vi "Alazar module U16.vi"(3 "Imag window array":sgl[](array[numeric]), 4 "Acq Settings":T2={"Window Type"=1, "Record Length"=1536, "Footer"=0, "Offset"=0, "Records Per Buffer"=1000, "Samples per record"=2048, "Records Count (Records/Acq)"=2147483647, "Output Format"=11} {"Output Format" items=["U16_LOG"=1, "U16_AMP2"=257]; "Window Type" items=["DSP_WINDOW_NONE", "DSP_WINDOW_HANNING", "DSP_WINDOW_HAMMING", "DSP_WINDOW_BLACKMAN", "DSP_WINDOW_BLACKMAN_HARRIS", "DSP_WINDOW_BARTLETT"]; "Footer" items=["FOOTER_NONE", "FOOTER_NPT"]}, 5 "Channel":u32(ring)=1 items=["A"=1, "B"=2, "A + B"=3, "C"=4, "A + C"=5, "A + B"=6, "D"=8, "A + D"=9, "B + D"=10, "C + D"=12, "A + B + C + D"=15], 6 "Trigger Settings":T5={"General Trigger Settings"={"Trigger Operation"=0, "Coupling ID"=2, "Range ID"=0, "Delay"=0, "Timeout Ticks"=0, "Mode"=0, "Parameter"=0}, "Trigger Engine 1"={"Trigger Engine"=0, "Source"=0, "Slope"=1, "Level"=0}, "Trigger Engine 2"={"Trigger Engine"=0, "Source"=0, "Slope"=1, "Level"=0}} {"General Trigger Settings"."Trigger Operation" items=["J", "K", "J OR K", "J AND K", "J XOR K", "J AND NOT K", "NOT J AND K"]; "General Trigger Settings"."Coupling ID" items=["AC"=1, "DC"=2]; "General Trigger Settings"."Range ID" items=["5 V", "1 V", "TTL"]; "Trigger Engine 1"."Trigger Engine" items=["J", "K"]; "Trigger Engine 1"."Source" items=["A", "B", "External", "Disable", "C", "D"]; "Trigger Engine 1"."Slope" items=["Positive"=1, "Negative"=2]; "Trigger Engine 2"."Trigger Engine" items=["J", "K"]; "Trigger Engine 2"."Source" items=["A", "B", "External", "Disable", "C", "D"]; "Trigger Engine 2"."Slope" items=["Positive"=1, "Negative"=2]}, 7 "Action":T1=enum."Config Trig", 8 "error in (no error)":errorcluster, 9 "Ch Input Control":T6={"Channel"=1, "Coupling"=2, "Range"=10, "Impedance"=2} {"Channel" items=["A"=1, "B"=2, "C"=4, "D"=8]; "Coupling" items=["AC"=1, "DC"=2]; "Range" items=["20 mV"=1, "40 mV"=2, "50 mV"=3, "80 mV"=4, "100 mV"=5, "200 mV"=6, "400 mV"=7, "500 mV"=8, "800 mV"=9, "1 V"=10, "1.25 V"=33, "2 V"=11, "4 V"=12, "5 V"=13, "8 V"=14, "10 V"=15, "20 V"=16]; "Impedance" items=["1 MOhm"=1, "50 Ohm"=2, ""=0]}, 10 "Capture Clock":T7={"Sample Rate"=30, "Decimation"=0, "Source"=1, "Edge"=0} {"Edge" items=["Rising", "Falling"]; "Source" items=["Internal"=1, "Fast External"=2, "Medium External"=3, "Slow External"=4, "External AC"=5, "External DC"=6, "External 10MHz"=7]}, 11 "Device ID":T8={"System ID"=1, "Board ID"=1}) -> (0 "error out":errorcluster, 1 "Return Code":u32, 2 "Buffer":u16[](array[numeric]))   [LabVIEW 2018]
uses:
  Hardware Mfg/AlazarTech SDK/Controls/Alazar Device ID.ctl
  Hardware Mfg/AlazarTech SDK/Controls/Clock Controls.ctl
  Hardware Mfg/AlazarTech SDK/Controls/Channel Input Controls.ctl
  Hardware Mfg/AlazarTech SDK/Controls/General Trigger Settings.ctl
  Hardware Mfg/AlazarTech SDK/Controls/Trigger Engine Controls.ctl
  Hardware Mfg/AlazarTech SDK/Controls/Alazar Acquisition Settings.ctl
  Hardware Mfg/AlazarTech SDK/Controls/Alazar Engine Actions.ctl
  Hardware Mfg/AlazarTech SDK/Controls/Async Read Parameters.ctl
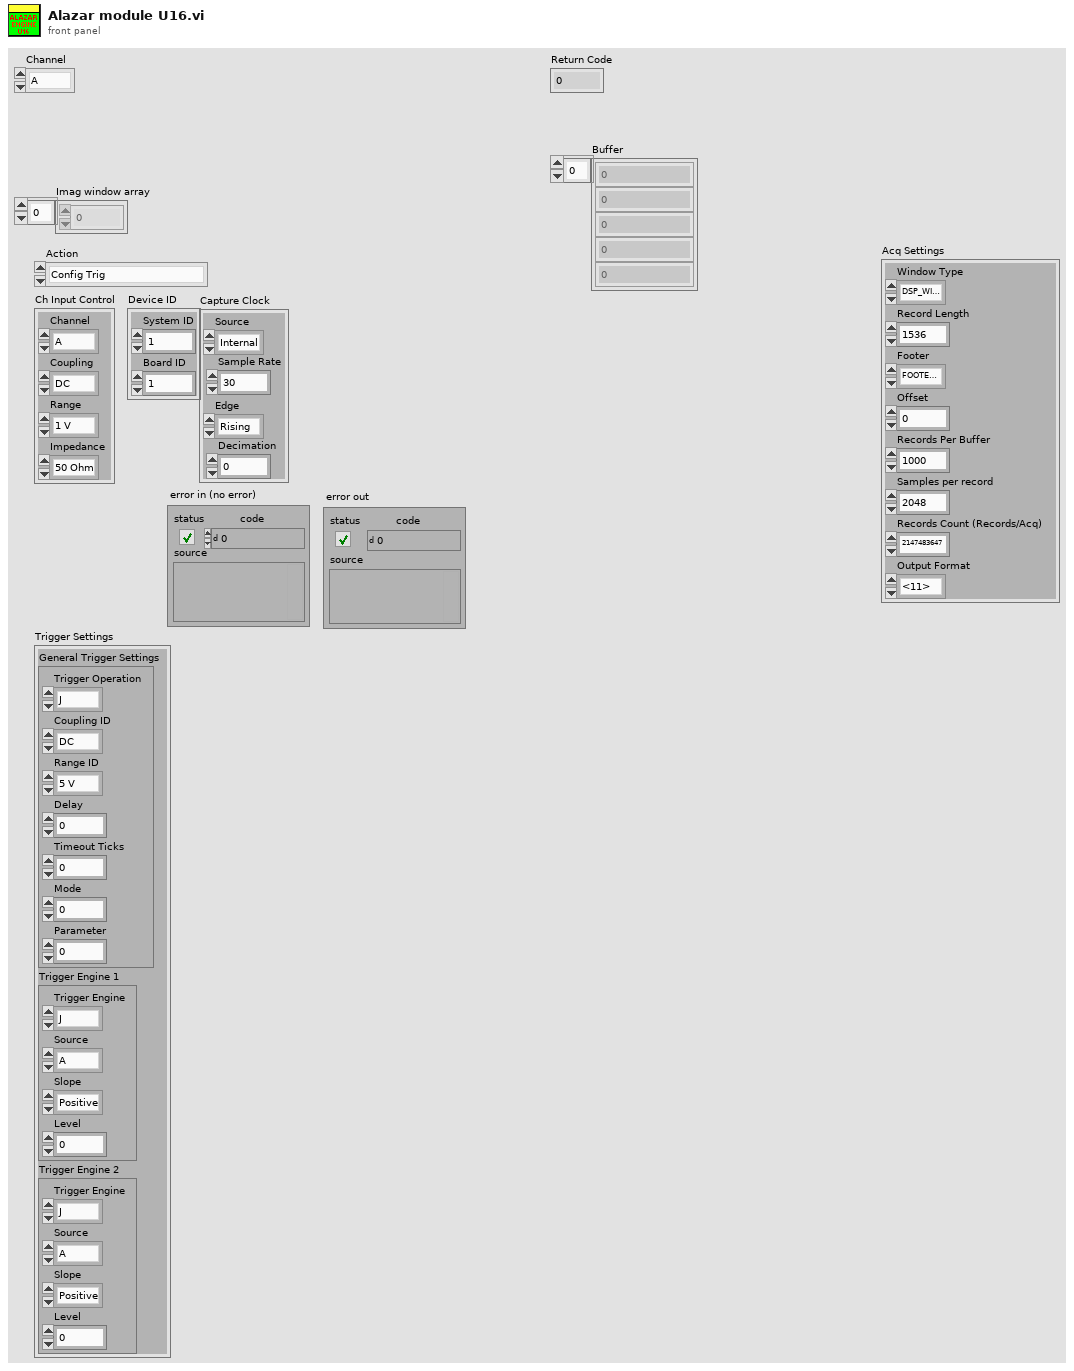
[diagram p1: front panel]
types:
  T1 = typedef "Alazar Engine Actions.ctl" = enum16{"Init", "Config Clock", "Config Ch", "Config Trig", "Config Non-FFT Acq.", "Non-FFT Acquire", "Load background from Non-FFT buffer", "enable background subtrac", "disable background subtrac", "load background from file", "load background from elsewhere", "start acquire", "background subtraction", "Config Acq.", "Acquire", "UnInit"}
  T2 = typedef "Alazar Acquisition Settings.ctl" = cluster{"Window Type":u32, "Record Length":u32, "Footer":u32, "Offset":u32, "Records Per Buffer":u32, "Samples per record":u32, "Records Count (Records/Acq)":u32, "Output Format":u32}
  T3 = typedef "General Trigger Settings.ctl" = cluster{"Trigger Operation":u32, "Coupling ID":u32, "Range ID":u32, "Delay":u32, "Timeout Ticks":u32, "Mode":u32, "Parameter":u32}
  T4 = typedef "Trigger Engine Controls.ctl" = cluster{"Trigger Engine":u32, "Source":u32, "Slope":u32, "Level":u32}
  T5 = cluster{"General Trigger Settings":T3, "Trigger Engine 1":T4, "Trigger Engine 2":T4}
  T6 = typedef "Channel Input Controls.ctl" = cluster{"Channel":u8, "Coupling":u32, "Range":u32, "Impedance":u32}
  T7 = typedef "Clock Controls.ctl" = cluster{"Sample Rate":u32, "Decimation":u32, "Source":u32, "Edge":u32}
  T8 = typedef "Alazar Device ID.ctl" = cluster{"System ID":u32, "Board ID":u32}
  T9 = typedef "Async Read Parameters.ctl" = cluster{"Transfer Offset":u32, "Transfer Length":u32, "Records Per Buffer":u32, "Records Per Acquisition":u32}
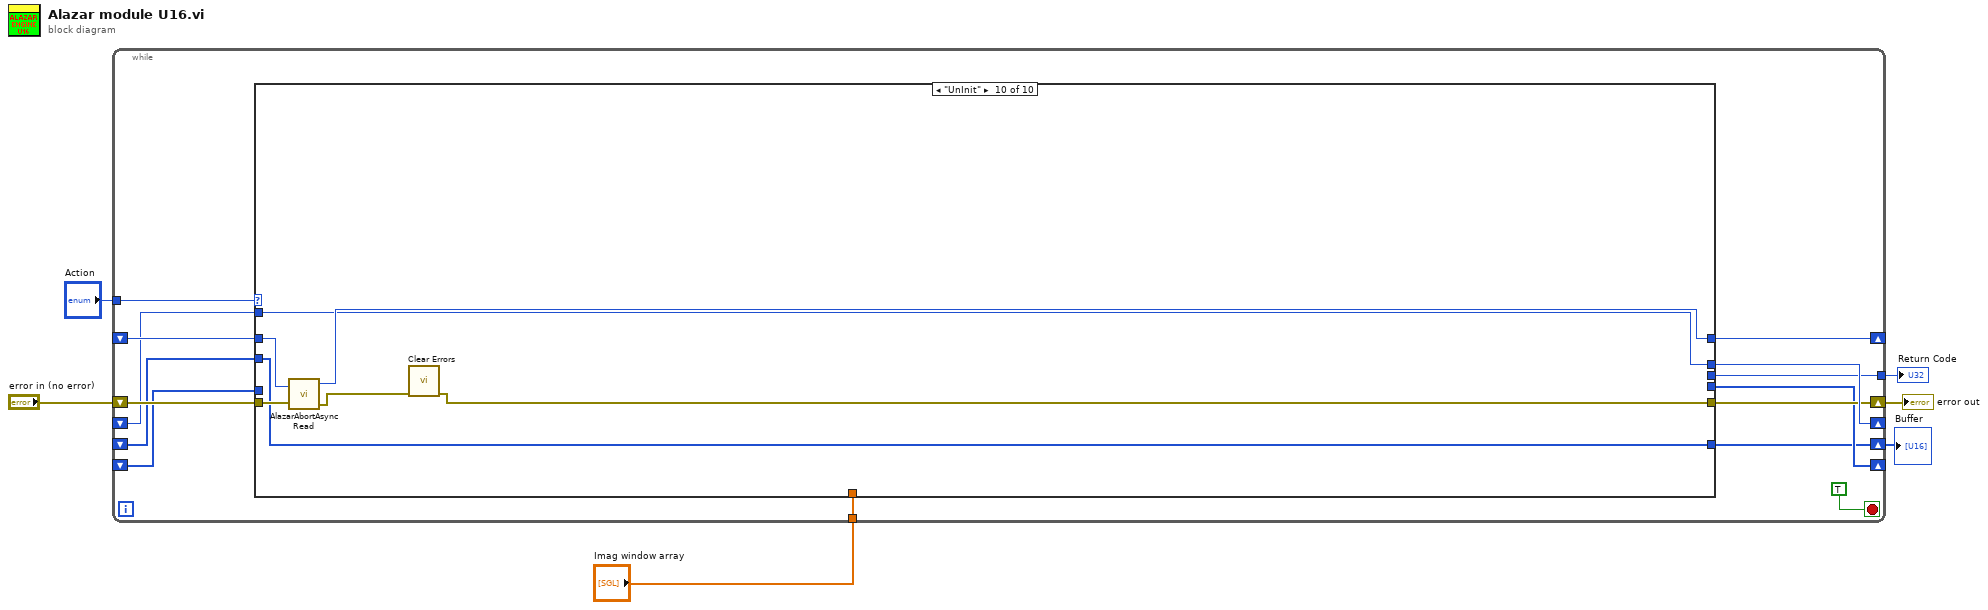
[diagram p0: block diagram]
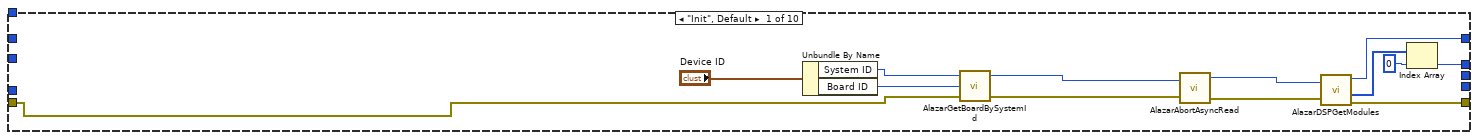
[diagram p2: hidden frame]
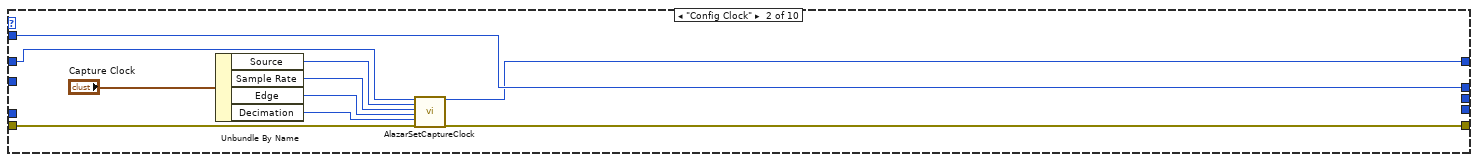
[diagram p3: hidden frame]
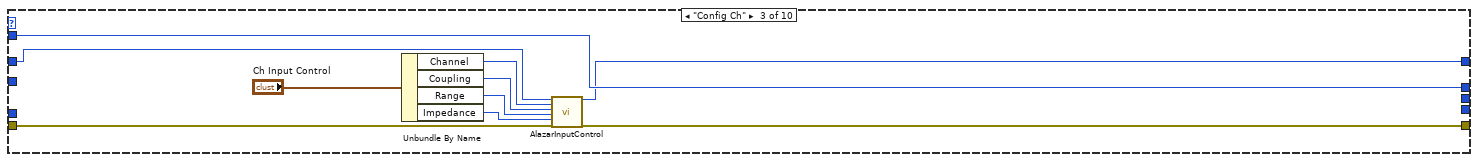
[diagram p4: hidden frame]
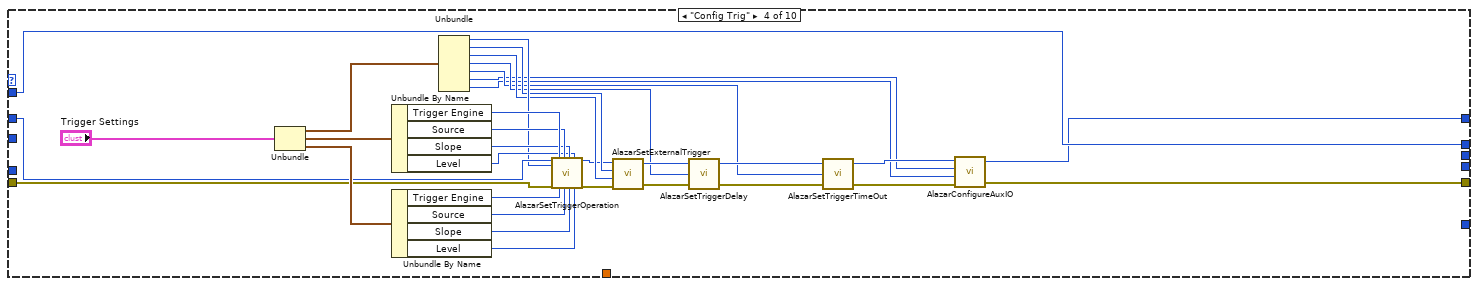
[diagram p5: hidden frame]
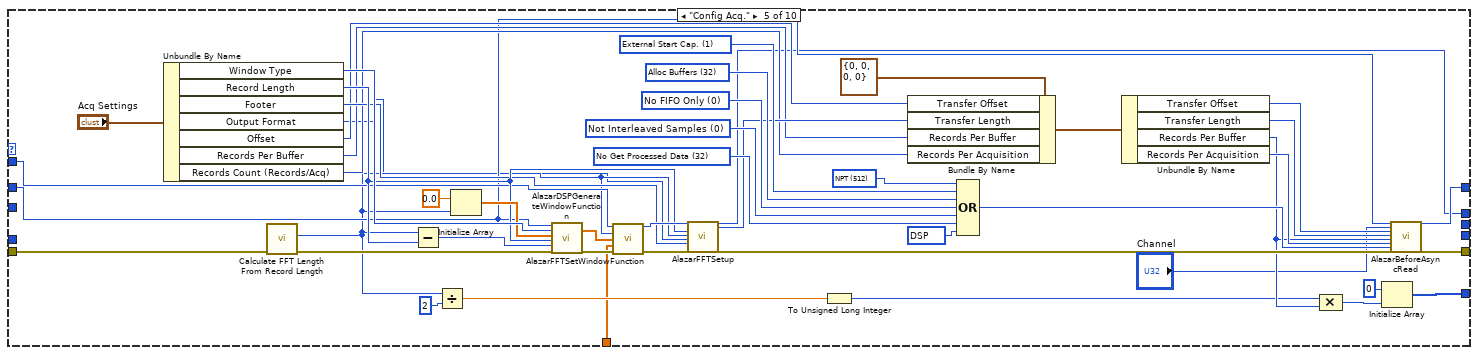
[diagram p6: hidden frame]
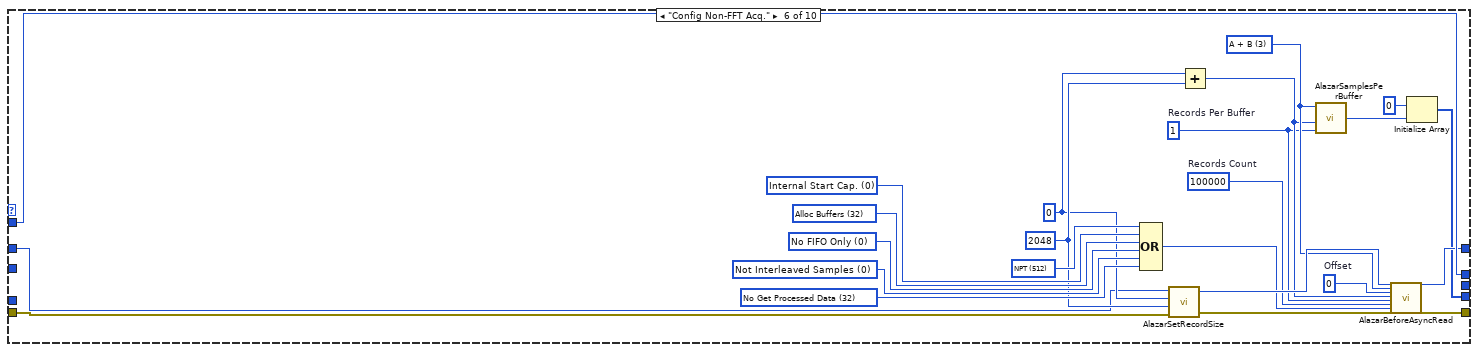
[diagram p7: hidden frame]
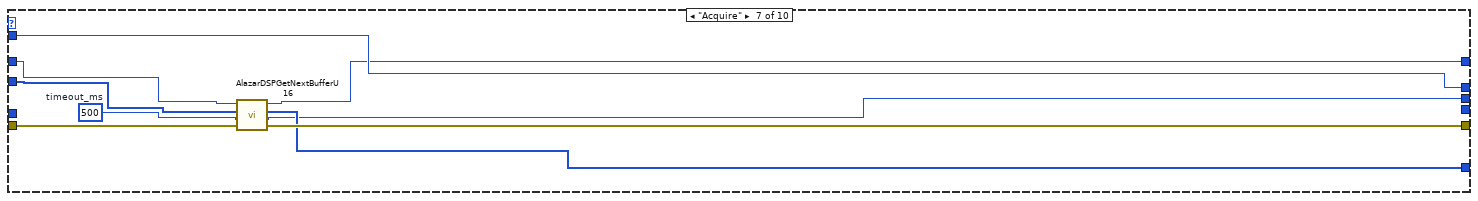
[diagram p8: hidden frame]
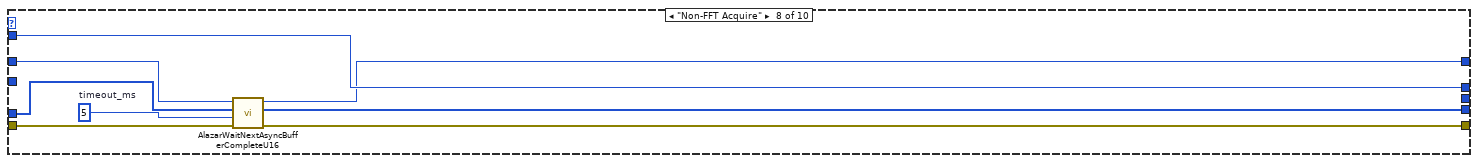
[diagram p9: hidden frame]
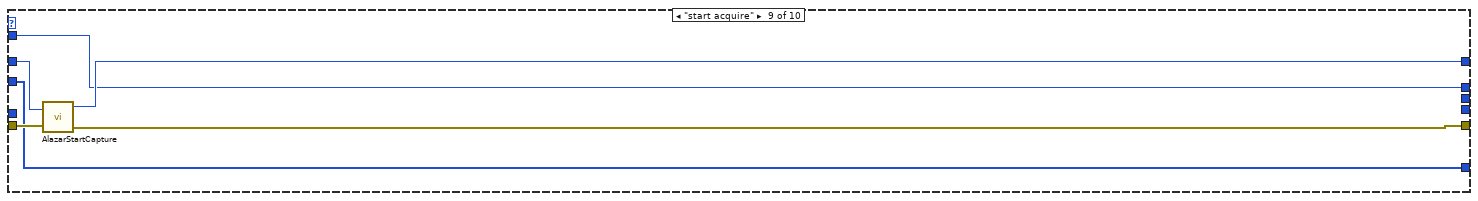
[diagram p10: hidden frame]
diagram:
  n1 = while {
    tunnel: "Action" -> [w18]
    shift-right: [w17] -> _
    shift-left: _ -> [w16]
    shift-right: [w15] -> _
    shift-left: _ -> [w14]
    shift-right: [w13] -> w4
    shift-left: "error in (no error)" -> [w19]
    shift-right: [w7] -> w1
    shift-left: _ -> [w12]
    shift-right: [w11] -> _
    shift-left: _ -> [w10]
    tunnel: "Imag window array" -> [w9]
    tunnel: [w8] -> w2
    stop <- TRUE stop-if-true
    n2 = case shown="\"UnInit\"" w18 {
      tunnel: w19 -> [w21 w41 w47 w67 w124 w138 w163 w170 w179 w186]
      tunnel: [w24 w34 w46 w55 w90 w137 w164 w167 w178 w180] -> w13
      tunnel: [w22 w35 w45 w54 w100 w134 w159 w168 w176 w184] -> w17
      tunnel: w16 -> [_ w36 w44 w72 w105 w136 w160 w171 w177 w185]
      tunnel: [w32 w43 w53 w83 w98 w135 w165 w169 w175 w183] -> w15
      tunnel: w14 -> [_ w43 w53 w83 w112 w135 w165 w169 w175 w183]
      tunnel: w12 -> [_ _ _ _ _ _ w161 _ w174 w181]
      tunnel: [_ _ _ _ _ w133 _ w166 _ _] -> w11
      tunnel: w10 -> [_ _ _ _ _ _ _ w172 _ _]
      tunnel: w9 -> [_ _ _ _ w88 _ _ _ _ _]
      tunnel: [_ _ _ _ _ _ w157 _ _ _] -> w8
      tunnel: [_ _ _ _ w87 _ w158 _ w174 w181] -> w7
      frame "Init", Default {
        n3 = Unbundle By Name("Device ID") -> ("System ID"=w30:u32, "Board ID"=w29:u32)
        n4 = call "AlazarGetBoardBySystemId.vi"("error in (no error)"=w21, "Board ID"=w29, "System ID"=w30) -> ("error out"=w28:errorcluster, "Handle"=w27:u64)  [unwired: 1 out]
        n5 = call "AlazarAbortAsyncRead.vi"("Handle"=w27, "error in (no error)"=w28) -> ("Handle"=w26:u64, "error out"=w25:errorcluster)  [unwired: 1 out]
        n6 = call "AlazarDSPGetModules.vi"("Handle"=w26, "error in (no error)"=w25) -> ("Handle"=w22:u64, "DSP Modules"=w23:u64[], "error out"=w24:errorcluster)  [unwired: 1 out]
        n7 = Index Array(array=w23, index=u32 0) -> (element=w32:u64)
      }
      frame "Config Clock" {
        n8 = Unbundle By Name("Capture Clock") -> ("Source"=w37:u32, "Sample Rate"=w38:u32, "Edge"=w39:u32, "Decimation"=w40:u32)
        n9 = call "AlazarSetCaptureClock.vi"("Handle"=w36, "Source"=w37, "Sample Rate"=w38, "Edge"=w39, "Decimation"=w40, "error in (no error)"=w41) -> ("Handle"=w35:u64, "error out"=w34:errorcluster)  [unwired: 11 in, 1 out]
      }
      frame "Config Ch" {
        n10 = Unbundle By Name("Ch Input Control") -> ("Channel"=w51:u8, "Coupling"=w50:u32, "Range"=w49:u32, "Impedance"=w48:u32)
        n11 = call "AlazarInputControl.vi"("Handle"=w44, "Channel"=w51, "Coupling"=w50, "Range"=w49, "Impedance"=w48, "error in (no error)"=w47) -> ("Handle"=w45:u64, "error out"=w46:errorcluster)  [unwired: 11 in, 1 out]
      }
      frame "Config Trig" {
        n12 = Unbundle("Trigger Settings") -> ("General Trigger Settings"=w84:T3, "Trigger Engine 1"=w82:T4, "Trigger Engine 2"=w81:T4)
        n13 = Unbundle By Name(w82) -> ("Trigger Engine"=w80:u32, "Source"=w79:u32, "Slope"=w78:u32, "Level"=w77:u32)
        n14 = Unbundle By Name(w81) -> ("Trigger Engine"=w76:u32, "Source"=w75:u32, "Slope"=w74:u32, "Level"=w73:u32)
        n15 = Unbundle(w84) -> ("Trigger Operation"=w71:u32, "Coupling ID"=w70:u32, "Range ID"=w69:u32, "Delay"=w63:u32, "Timeout Ticks"=w60:u32, "Mode"=w57:u32, "Parameter"=w56:u32)
        n16 = call "AlazarSetTriggerOperation.vi"("Handle"=w72, "Trigger Operation"=w71, "error in (no error)"=w67, "Trigger Engine 1"=w80, "Trigger Engine 2"=w76, "Source 1"=w79, "Source 2"=w75, "Slope 1"=w78, "Slope 2"=w74, "Level 1"=w77, "Level 2"=w73) -> ("Handle"=w65:u64, "error out"=w68:errorcluster)  [unwired: 6 in, 1 out]
        n17 = call "AlazarSetExternalTrigger.vi"("error in (no error)"=w68, "Range ID"=w69, "Coupling ID"=w70, "Handle"=w65) -> ("error out"=w66:errorcluster, "Handle"=w64:u64)  [unwired: 1 out]
        n18 = call "AlazarSetTriggerDelay.vi"("error in (no error)"=w66, "Delay"=w63, "Handle"=w64) -> ("error out"=w62:errorcluster, "Handle"=w61:u64)  [unwired: 1 out]
        n19 = call "AlazarSetTriggerTimeOut.vi"("error in (no error)"=w62, "Timeout Ticks"=w60, "Handle"=w61) -> ("error out"=w59:errorcluster, "Handle"=w58:u64)  [unwired: 1 out]
        n20 = call "AlazarConfigureAuxIO.vi"("error in (no error)"=w59, "Parameter"=w56, "Mode"=w57, "Handle"=w58) -> ("error out"=w55:errorcluster, "Handle"=w54:u64)  [unwired: 1 out]
      }
      frame "Config Acq." {
        w125 = u32 16384 items=["DSP"=16384]
        w131 = u32 32 items=["No Get Processed Data"=32, "Get Processed Data"=8192]
        w130 = u32 0 items=["Not Interleaved Samples"=0, "Interleave Samples"=4096]
        w126 = u32 0 items=["No FIFO Only"=0, "FIFO Only"=2048]
        w129 = u32 32 items=["Alloc Buffers"=32]
        w128 = u32 1 items=["Internal Start Cap.", "External Start Cap."]
        w127 = u32 512 items=["Traditional"=0, "NPT"=512, "Continuous"=256, "Triggered Streaming"=1024]
        n21 = Unbundle By Name("Acq Settings") -> ("Window Type"=w121:u32, "Record Length"=w115:u32, "Footer"=w114:u32, "Output Format"=w86:u32, "Offset"=w110:u32, "Records Per Buffer"=w108:u32, "Records Count (Records/Acq)"=w107:u32)
        n22 = call "Calculate FFT Length From Record Length.vi"("error in (no error)"=w124) -> ("error out"=w122:errorcluster, "FFT Length"=w96:u32)  [unwired: 8 in, 1 out]
        n23 = Subtract(x=w96, y=w115) -> (x-y=w120:u32)
        n24 = Divide(x=w96, y=u32 2) -> (x/y=w92:dbl)
        n25 = Initialize Array(sgl 0.0, w96) -> (w118:sgl[])
        n26 = call "AlazarDSPGenerateWindowFunction.vi"("Handle"=w105, "Window Type"=w121, "window"=w118, "WindowLength_samples"=w115, "PaddingLength_samples"=w120, "error in (no error)"=w122) -> ("window"=w119:sgl[], "error out"=w117:errorcluster)  [unwired: 10 in, 2 out]
        n27 = call "AlazarFFTSetWindowFunction.vi"("DSP Handle"=w112, "Samples per record"=w96, "Real window array"=w119, "Imag window array"=w88, "error in (no error)"=w117) -> ("DSP Handle"=w116:u64, "error out"=w113:errorcluster)  [unwired: 9 in]
        n28 = call "AlazarFFTSetup.vi"("DSP Handle"=w116, "Record Length (samples)"=w115, "FFT Length (samples)"=w96, "Output Format"=w86, "Footer"=w114, "error in (no error)"=w113) -> ("DSP Handle"=w98:u64, "Bytes Per Output Record"=w109:u32, "error out"=w99:errorcluster)  [unwired: 18 in, 1 out]
        n29 = To Unsigned Long Integer(number=w92) -> (unsigned 32bit integer=w91:u32)
        n30 = Bundle By Name(cluster=T9 {"Transfer Offset"=0, "Transfer Length"=0, "Records Per Buffer"=0, "Records Per Acquisition"=0} ("ASync Read Parameters"), "Transfer Offset"=w110, "Transfer Length"=w109, "Records Per Buffer"=w108, "Records Per Acquisition"=w107) -> (w106:T9)
        n31 = Compound Arithmetic op=OR(w127, w128, w129, w126, w130, w131, w125) -> (w101:u32)
        n32 = Unbundle By Name(w106) -> ("Transfer Offset"=w104:u32, "Transfer Length"=w103:u32, "Records Per Buffer"=w97:u32, "Records Per Acquisition"=w102:u32)
        n33 = Compound Arithmetic op=MULTIPLY(w91, w97) -> (w95:u32)
        n34 = Initialize Array(u16 0 ("element"), w95) -> (w87:u16[])
        n35 = call "AlazarBeforeAsyncRead.vi"("Handle"=w105, "Channel Select"="Channel", "Transfer Offset"=w104, "Transfer Length"=w103, "Records Per Buffer"=w97, "Records Per Acquisition"=w102, "Flags"=w101, "error in (no error)"=w99) -> ("Handle"=w100:u64, "error out"=w90:errorcluster)  [unwired: 17 in, 1 out]
      }
      frame "Config Non-FFT Acq." {
        w141 = u32 3 items=["A"=1, "B"=2, "A + B"=3, "C"=4, "A + C"=5, "A + B"=6, "D"=8, "A + D"=9, "B + D"=10, "C + D"=12, "A + B + C + D"=15] ("Channel 2")
        w144 = u32 100000  # Records Count
        w139 = u32 1  # Records Per Buffer
        w145 = u32 0  # Offset
        w150 = u32 2048 ("Post-trigger Samples")
        w149 = u32 0 ("Pre-trigger Samples")
        w156 = u32 32 items=["No Get Processed Data"=32, "Get Processed Data"=8192]
        w155 = u32 0 items=["Not Interleaved Samples"=0, "Interleave Samples"=4096]
        w151 = u32 0 items=["No FIFO Only"=0, "FIFO Only"=2048]
        w154 = u32 32 items=["Alloc Buffers"=32]
        w153 = u32 0 items=["Internal Start Cap.", "External Start Cap."]
        w152 = u32 512 items=["Traditional"=0, "NPT"=512, "Continuous"=256, "Triggered Streaming"=1024]
        n36 = Compound Arithmetic op=OR(w152, w153, w154, w151, w155, w156) -> (w146:u32)
        n37 = call "AlazarSetRecordSize.vi"("error in (no error)"=w138, "Post-trigger Samples"=w150, "Pre-trigger Samples"=w149, "Handle"=w136) -> ("error out"=w147:errorcluster, "Handle"=w148:u64)  [unwired: 1 out]
        n38 = Add(x=w149, y=w150) -> (x+y=w140:u32)
        n39 = call "AlazarSamplesPerBuffer.vi"("Records Per Buffer"=w139, "Samples Per Record"=w140, "Channel Mask"=w141) -> ("Samples Per Buffer"=w142:u32)  [unwired: 1 in]
        n40 = call "AlazarBeforeAsyncRead.vi"("Handle"=w148, "Channel Select"=w141, "Transfer Offset"=w145, "Transfer Length"=w140, "Records Per Buffer"=w139, "Records Per Acquisition"=w144, "Flags"=w146, "error in (no error)"=w147) -> ("Handle"=w134:u64, "error out"=w137:errorcluster)  [unwired: 17 in, 1 out]
        n41 = Initialize Array(u16 0, w142) -> (w133:u16[])
      }
      frame "Acquire" {
        w162 = u32 500  # timeout_ms
        n42 = call "AlazarDSPGetNextBufferU16.vi"("error in (no error)"=w163, "timeout_ms"=w162, "Buffer"=w161, "Handle"=w160) -> ("error out"=w164:errorcluster, "Return Code"=w157:u32, "Buffer"=w158:u16[], "Handle"=w159:u64)
      }
      frame "Non-FFT Acquire" {
        w173 = u32 5  # timeout_ms
        n43 = call "AlazarWaitNextAsyncBufferCompleteU16.vi"("error in (no error)"=w170, "Timeout (ms)"=w173, "Buffer"=w172, "Handle"=w171) -> ("error out"=w167:errorcluster, "Buffer"=w166:u16[], "Handle"=w168:u64)  [unwired: 1 out]
      }
      frame "start acquire" {
        n44 = call "AlazarStartCapture.vi"("Handle"=w177, "error in (no error)"=w179) -> ("Handle"=w176:u64, "error out"=w178:errorcluster)  [unwired: 1 out]
      }
      frame "UnInit" {
        n45 = call "AlazarAbortAsyncRead.vi"("Handle"=w185, "error in (no error)"=w186) -> ("Handle"=w184:u64, "error out"=w182:errorcluster)  [unwired: 1 out]
        n46 = call <vilib>:"Clear Errors.vi"("error in (no error)"=w182) -> ("error out"=w180:errorcluster)  [unwired: 5 in, 1 out]
      }
    }
  }
  "error out" <- w4
  "Buffer" <- w1
  "Return Code" <- w2
